vi "Test_PublishCluster_SubBeforePub_OK.vi"(8 "error in (no error)":errorcluster, 11 "TestMediator In":refnum<class "TestMediator.lvclass">) -> (0 "error out":errorcluster, 3 "TestMediator Out":refnum<class "TestMediator.lvclass">)   [LabVIEW 2015, in "TestMediator.lvclass"]
uses:
  TestMediator.lvclass
  Mediator/Mediator.lvclass
  Transport/QueueTransport/QueueTransport.lvclass/QueueTransport.ctl
  SubscriptionPolicy/BasicSubscription/BasicSubscription.lvclass/BasicSubscription.ctl
  IMediator/SubscriptionRequest/SubscriptionRequest.lvclass/SubscriptionRequest.ctl
  IMediator/IMediator Messages/Subscribe Msg/Subscribe Msg.lvclass/Subscribe Msg.ctl
  <vilib>/ActorFramework/Message Enqueuer/Message Enqueuer.lvclass/Message Enqueuer.ctl
  IMediator/IMediator Messages/Publish Msg/Publish Msg.lvclass/Publish Msg.ctl
  <vilib>/ActorFramework/Message Enqueuer/Enqueue.vi
  <vilib>/Utility/error.llb/Error Cluster From Error Code.vi
  <vilib>/ActorFramework/Message Priority Queue/Priority Enqueue.vi
  SubscriptionPolicy/BasicSubscription/BasicSubscription.lvclass
  Transport/QueueTransport/QueueTransport.lvclass
  IMediator/SubscriptionRequest/SubscriptionRequest.lvclass
  IMediator/IMediator Messages/Subscribe Msg/Subscribe Msg.lvclass
  IMediator/IMediator Messages/Publish Msg/Publish Msg.lvclass
  <vilib>/ActorFramework/Stop Msg/Stop Msg.lvclass
  <vilib>/addons/_JKI Toolkits/VI Tester/TestCase.llb/TestCase.lvclass
  <vilib>/ActorFramework/Actor/Actor.lvclass
  IMediator/ISubscriptionPolicy/ISubscriptionPolicy.lvclass
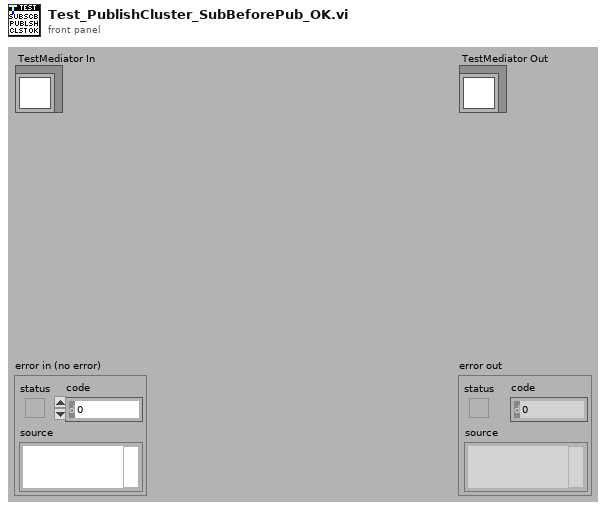
[diagram p1: front panel]
types:
  T1 = typedef "IMediator.lvlib/ISubscriptionPolicy.lvclass/ISubscriptionPolicy Reference.ctl" = refnum<data-value>
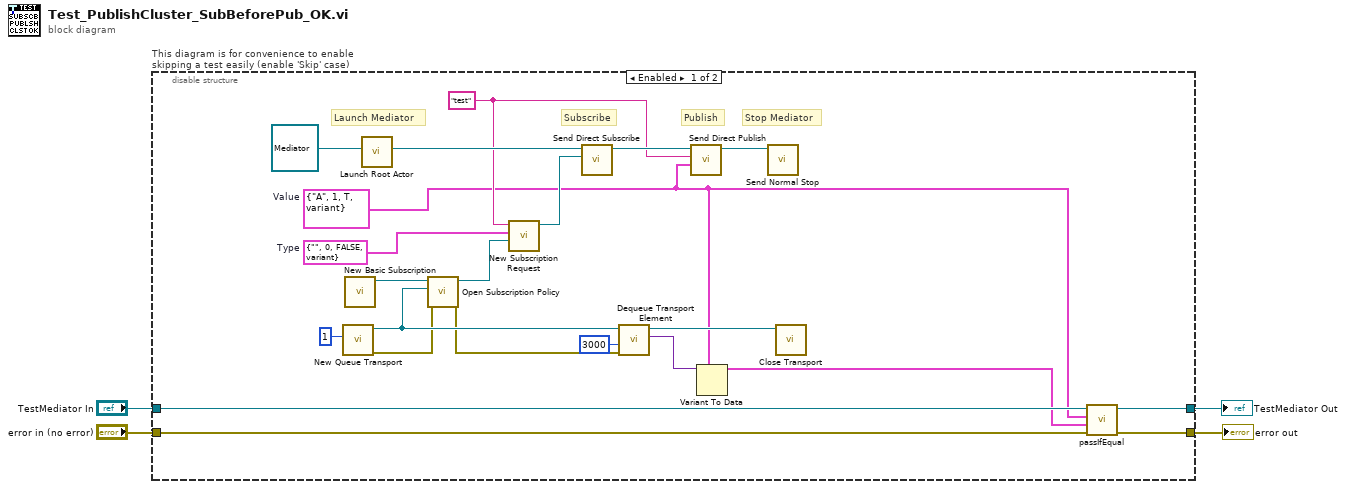
[diagram p0: block diagram]
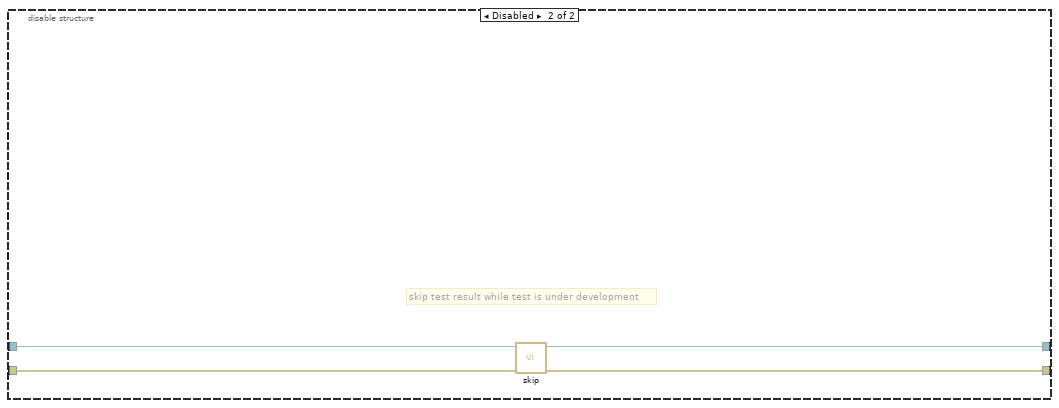
[diagram p2: hidden frame]
diagram:
  n1 = disable-structure "This diagram is for convenience to enable skipping a test easily (enable 'Skip' case)" shown="Enabled" {
    disable-tunnel: "TestMediator In" -> [w26 w30]
    disable-tunnel: [w25 w28] -> w1
    disable-tunnel: [w24 w29] -> w3
    disable-tunnel: "error in (no error)" -> [w23 w27]
    frame Enabled {
      w6 = cluster{string, i32, bool, variant} {"", 0, FALSE, variant}  # Type
      w7 = cluster{string, i32, bool, "variant":variant} {"A", 1, TRUE, "variant"=variant(i32 2)}  # Value
      w8 = "test" ("Datum Name")
      # "Launch Mediator"
      # "Stop Mediator"
      # "Subscribe"
      # "Publish"
      n2 = call "New Queue Transport.vi"("Max Queue Size (-1)"=1) -> ("error out"=w17:errorcluster, "QueueTransport"=w19:refnum<class "QueueTransport.lvclass">)  [unwired: 9 in]
      n3 = call "New Basic Subscription.vi"() -> ("BasicSubscription Out"=w12:refnum<class "BasicSubscription.lvclass">)  [unwired: 11 in]
      n4 = call <vilib>:"Launch Root Actor.vi"("Actor"=refnum<class "Mediator.lvclass"> refnum ("Mediator.lvlib:Mediator.lvclass")) -> ("Actor's Enqueuer"=w9:refnum<class "Message Enqueuer.lvclass">)  [unwired: 9 in, 1 out]
      n5 = call "Open Subscription Policy.vi"("error in (no error)"=w17, "Transport"=w19, "SubscriptionPolicy"=w12) -> ("error out"=w16:errorcluster, "Subscription Policy"=w5:T1)  [unwired: 7 in]
      n6 = call "New Subscription Request.vi"("Subscription Policy"=w5, "Type"=w6, "Datum Name"=w8) -> ("SubscriptionRequest"=w21:refnum<class "SubscriptionRequest.lvclass">)  [unwired: 8 in]
      n7 = call "Send Direct Subscribe.vi"("Subscription Request"=w21, "Message Enqueuer"=w9) -> ("Message Enqueuer out"=w11:refnum<class "Message Enqueuer.lvclass">)  [unwired: 8 in, 1 out]
      n8 = call "Dequeue Transport Element.vi"("error in (no error)"=w16, "Timeout In ms (-1)"=3000, "QueueTransport in"=w19) -> ("Data"=w14:variant, "QueueTransport out"=w15:refnum<class "QueueTransport.lvclass">)  [unwired: 5 in, 2 out]
      n9 = call "Send Direct Publish.vi"("Data to Publish"=w7, "Datum Name"=w8, "Mediator Enqeuer"=w11) -> ("Mediator Enqueuer out"=w10:refnum<class "Message Enqueuer.lvclass">)  [unwired: 7 in, 1 out]
      n10 = Variant To Data(type=w7, Variant=w14) -> (data=w13:cluster{string, i32, bool, "variant":variant})  [unwired: 1 in, 1 out]
      n11 = call <vilib>:"Send Normal Stop.vi"("Message Enqueuer"=w10) -> ()  [unwired: 10 in, 1 out]
      n12 = call-dynamic "Close Transport.vi"("QueueTransport in"=w15) -> ()  [unwired: 10 in, 1 out]
      n13 = call-dynamic "passIfEqual.vi"("error in (no error)"=w23, "y"=w13, "x"=w7, "TestCase in"=w26) -> ("error out"=w24:errorcluster, "TestCase out"=w25:refnum<class "TestMediator.lvclass">)  [unwired: 6 in]
    }
    frame Disabled {
      # "skip test result while test is under development"
      n14 = call <vilib>:"skip.vi"("error in (no error)"=w27, "TestCase in"=w30) -> ("error out"=w29:errorcluster, "TestCase out"=w28:refnum<class "TestMediator.lvclass">)  [unwired: 8 in]
    }
  }
  "error out" <- w3
  "TestMediator Out" <- w1
